vi "Norm.vi"(8 "error in (no error)":errorcluster, 10 "2D vector":dbl[](array[numeric]), 11 "Utilities in":refnum<class "Utilities.lvclass">) -> (0 "error out":errorcluster, 2 "Modulo":dbl, 3 "Utilities out":refnum<class "Utilities.lvclass">)   [LabVIEW 2023, in "Utilities.lvclass"]
uses:
  Utilities.lvclass
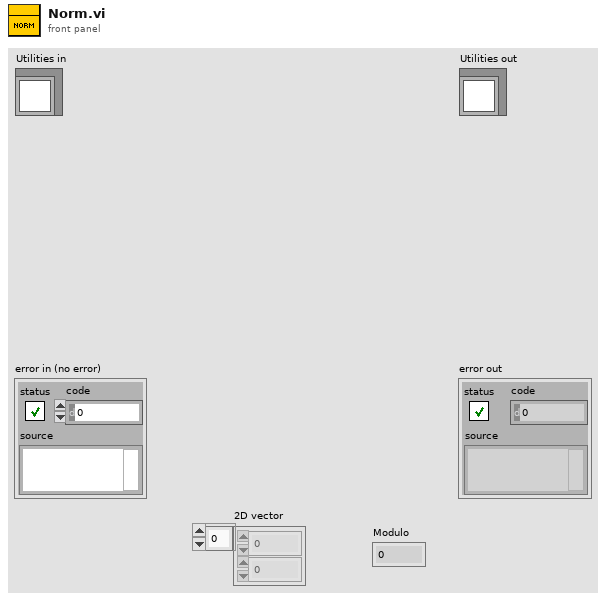
[diagram p1: front panel]
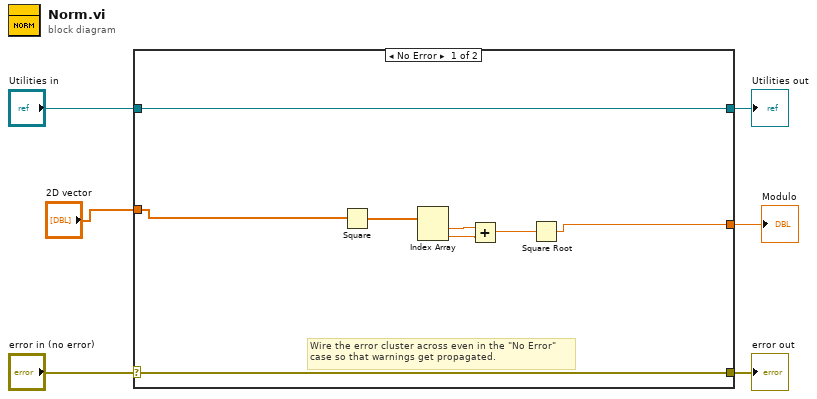
[diagram p0: block diagram]
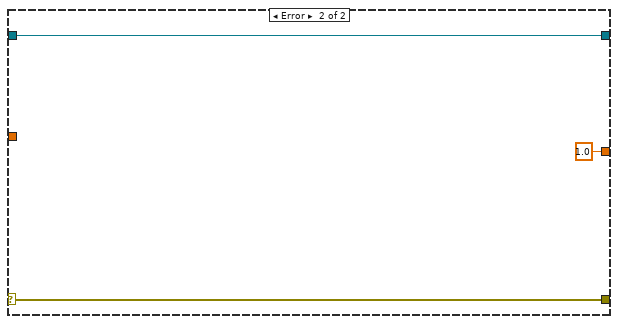
[diagram p2: hidden frame]
diagram:
  n1 = case shown="No Error" "error in (no error)" {
    selector: "error in (no error)" -> [w13 w17]
    tunnel: [w13 w17] -> w5
    tunnel: [w14 w16] -> w3
    tunnel: "Utilities in" -> [w14 w16]
    tunnel: "2D vector" -> [w9 _]
    tunnel: [w7 1.0] -> w1
    frame No Error {
      # "Wire the error cluster across even in the \"No Error\"\ncase so that warnings get propagated."
      n2 = Square(x=w9) -> (x^2=w12:dbl[])
      n3 = Index Array(array=w12) -> (element #1=w11:dbl, element #2=w10:dbl)  [unwired: 2 in]
      n4 = Add(x=w11, y=w10) -> (x+y=w8:dbl)
      n5 = Square Root(x=w8) -> (sqrt(x)=w7:dbl)
    }
    frame Error {
    }
  }
  "error out" <- w5
  "Utilities out" <- w3
  "Modulo" <- w1
